vi "LoadNewLevel.vi"(8 "error in (no error)":errorcluster, 11 "Bouncer in":refnum<class "Bouncer.lvclass">) -> (0 "error out":errorcluster, 3 "Bouncer out":refnum<class "Bouncer.lvclass">)   [LabVIEW 2019, in "RT_Game.lvlib" / "Bouncer.lvclass"]
uses:
  Bouncer.lvclass
  C:/Users/FreshBob/Dropbox/VIs/myRIO_GameConsole/RT/RT_Game/Game/Game.lvclass
  Menu/States.ctl
  Game/Game.lvclass/Game.ctl
  Bouncer.lvclass/Bouncer.ctl
  Game/Read State.vi
  PongBall/PongBall.lvclass
  Game/Game.lvclass
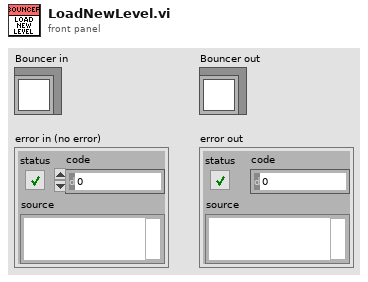
[diagram p1: front panel]
types:
  T1 = typedef "RT_Game.lvlib/Game.lvclass/States.ctl" = enum16{"Init", "Restart", "Menu", "Game", "Resume", "ToggleSingleplayer", "LoadNextGame", "ExitToMenu", "NewHighscore", "GameOver", "SlideOut"}
  T2 = enum16{"all", "up", "down", "left", "right", "leftup", "rightup", "leftdown", "rightdown"}
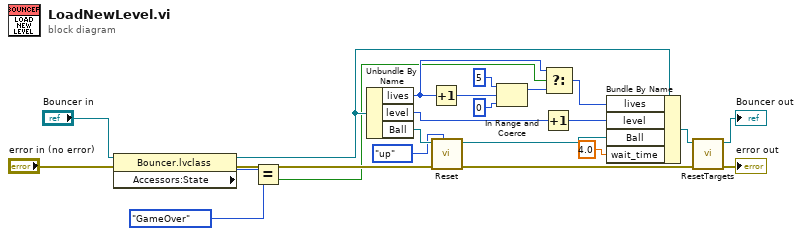
[diagram p0: block diagram]
diagram:
  n1 = property class="Bouncer.lvclass"(reference="Bouncer in", error in="error in (no error)") -> (reference out=w6:refnum<class "Bouncer.lvclass">, error out=w8:errorcluster, "Accessors:State"=w4:T1)
  n2 = Equal?(x=w4, y=States."GameOver" ("x")) -> (x = y?=w2:bool)
  n3 = Unbundle By Name(w6) -> ("lives"=w3:i16, "level"=w15:i16, "Ball"=w21:refnum<class "PongBall.lvclass">)
  n4 = Increment(x=w3) -> (x+1=w12:i16)
  n5 = call "Reset.vi"("Direction (all)"=T2."up", "error in (no error)"=w8, "PongBall in"=w21) -> ("error out"=w20:errorcluster, "PongBall out"=w22:refnum<class "PongBall.lvclass">)  [unwired: 7 in]
  n6 = In Range and Coerce(upper limit=i16 5, x=w12, lower limit=i16 0) -> (coerced(x)=w11:i16)  [unwired: 1 out]
  n7 = Increment(x=w15) -> (x+1=w14:i16)
  n8 = Select(t=w3, s=w2, f=w11) -> (s? t:f=w5:i16)
  n9 = Bundle By Name(cluster=w6, "lives"=w5, "level"=w14, "Ball"=w22, "wait_time"=4.0) -> (w17:refnum<class "Bouncer.lvclass">)
  n10 = call "ResetTargets.vi"("error in (no error)"=w20, "Bouncer in"=w17) -> ("error out"=→"error out":errorcluster, "Bouncer out"=→"Bouncer out":refnum<class "Bouncer.lvclass">)  [unwired: 8 in]
